vi "Disable Front Panel Updates.vi"(7 "VI Refnum":refnum<vi>, 10 "error in (no error)":errorcluster, 11 "Disable?":bool) -> (2 "error out":errorcluster)   [LabVIEW 2016, in "Assert API Components.lvlib" / "Assert Display.lvlib" / "Main Display.lvlib" / "Main Display.lvclass"]
uses:
  Main Display.lvclass
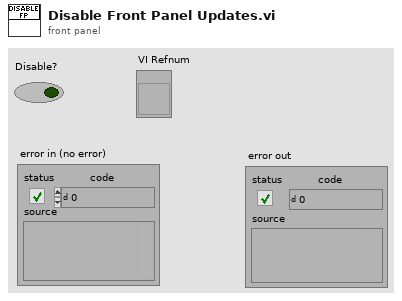
[diagram p1: front panel]
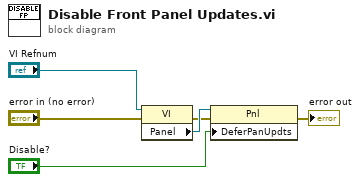
[diagram p0: block diagram]
diagram:
  n1 = property class="VI"(reference="VI Refnum", error in="error in (no error)") -> (error out=w4:errorcluster, "Panel"=w5:refnum<vi>)  [unwired: 1 out]
  n2 = property class="Pnl"(reference=w5, error in=w4, "DeferPanUpdts"="Disable?") -> (error out=→"error out":errorcluster)  [unwired: 1 out]
